vi "DevTests_ExeTTF.vi"() -> ()   [LabVIEW 2026]
uses:
  SDL3/Error/GetError-UiThread.vi
  SDL3/Error/GetError-AnyThread.vi
  <vilib>/Utility/error.llb/Error Cluster From Error Code.vi
  SDL3/Init/Init.lvlib
  SDL3/TTF/TTF.lvlib
panel:
  out "error out":errorcluster
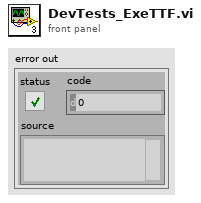
[diagram p1: front panel]
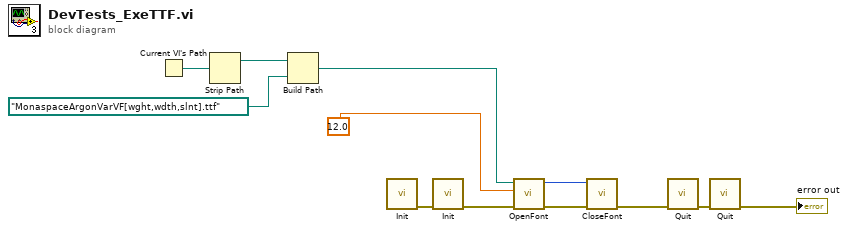
[diagram p0: block diagram]
diagram:
  n1 = Current VI's Path() -> (path=w5:path)
  n2 = Strip Path(path=w5) -> (stripped path=w4:path)  [unwired: 1 out]
  n3 = Build Path(base path=w4, name or relative path=path "MonaspaceArgonVarVF[wght,wdth,slnt].ttf") -> (appended path=w2:path)
  n4 = call "Init.vi"() -> ("error out"=w12:errorcluster)  [unwired: 11 in]
  n5 = call "Init.vi"("No Error"=w12) -> ("error out"=w9:errorcluster)  [unwired: 10 in]
  n6 = call "OpenFont.vi"("No Error"=w9, "Pt Size"=sgl 12.0, "File"=w2) -> ("error out"=w8:errorcluster, "Font [TTF_Font *]"=w6:i64)  [unwired: 7 in]
  n7 = call "CloseFont.vi"("No Error"=w8, "Font [TTF_Font *]"=w6) -> ("error out"=w7:errorcluster)  [unwired: 9 in]
  n8 = call "Quit.vi"("No Error"=w7) -> ("error out"=w11:errorcluster)  [unwired: 10 in]
  n9 = call "Quit.vi"("No Error"=w11) -> ("error out"=→"error out":errorcluster)  [unwired: 10 in]
